vi "GlobalVariable.vi"() -> ()   [LabVIEW 2017]
panel:
  out "colorCubeArray":dbl[](array[numeric])
  out "colorBoxArray":dbl[](array[numeric])
  in  "colorEnum":T1(ring)
  out "3CoordinateBox":dbl[](array[numeric])
  out "2CoordinateBox":dbl[](array[numeric])
  out "1CoordinateBox":dbl[](array[numeric])
  out "colorArray":dbl[](array[numeric])
  # "0 center x"
  # "1 center y"
  # "2 left"
  # "3 up"
  # "4 right"
  # "5 bot"
  # "6 width"
  # "7 height"
  # "8 tayang"
  # "9 area"
  # "10 convex hull area"
  # "11 img area"
  # "12 %area/img area"
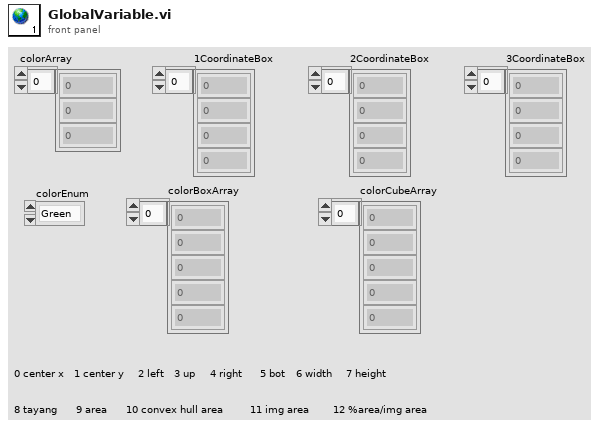
[diagram p1: front panel]
types:
  T1 = enum16{"Green", "Yellow", "Red", "Blue", "Orange", "Null"}
diagram:
